vi "Apparent Wind RP.vi"() -> (0 "Apparent Wind Direction RP":dbl, 1 "Apparent Wind Direction RP ABS":dbl, 2 "Apparent Wind Speed RP ABS":dbl, 3 "Apparent Wind Speed RP":dbl)   [LabVIEW 2011]
doc: "This VI replaces all Apparent Wind and Absolute Wind Reads. Only the wind records VI is using the actual sensor values.\nThe outputs are wind direction and speed, absolute and apparent (absolute indicated with ABS in the output's name)."
uses:
  2 Globals/2 Global.vi
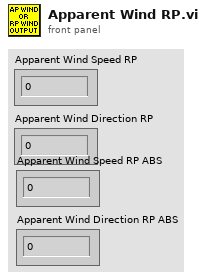
[diagram p1: front panel]
types:
  T1 = typedef "apparent wind direction.ctl" = dbl
  T2 = typedef "absolute wind direction.ctl" = dbl
  T3 = typedef "absolute wind speed.ctl" = dbl
  T4 = typedef "apparent wind speed.ctl" = dbl
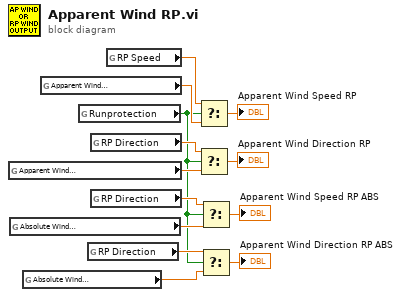
[diagram p0: block diagram]
diagram:
  n1 = global read "2 Global.vi" "Apparent Wind\nDirection (º)"() -> (w10:T1)
  n2 = global read "2 Global.vi" "Absolute Wind\nDirection (º)"() -> (w3:T2)
  n3 = global read "2 Global.vi" "Absolute Wind\nSpeed"() -> (w4:T3)
  n4 = global read "2 Global.vi" "Apparent Wind\nSpeed"() -> (w11:T4)
  n5 = global read "2 Global.vi" "Runprotection"() -> (w1:bool)
  n6 = global read "2 Global.vi" "RP Direction"() -> (w2:T1)
  n7 = global read "2 Global.vi" "RP Direction"() -> (w12:T1)
  n8 = global read "2 Global.vi" "RP Direction"() -> (w5:T1)
  n9 = global read "2 Global.vi" "RP Speed"() -> (w13:T4)
  n10 = Select(t=w13, s=w1, f=w11) -> (s? t:f=→"Apparent Wind Speed RP":T4)
  n11 = Select(t=w12, s=w1, f=w10) -> (s? t:f=→"Apparent Wind Direction RP":T1)
  n12 = Select(t=w5, s=w1, f=w3) -> (s? t:f=→"Apparent Wind Speed RP ABS":T2)
  n13 = Select(t=w2, s=w1, f=w4) -> (s? t:f=→"Apparent Wind Direction RP ABS":T3)
